vi "IPC-Modbus-Transfer-EncodeResponse-ReadCoils.vi"(11 "Coil Status":bool[](array[boolean])) -> (3 "输出字符串":string)   [LabVIEW 2014]
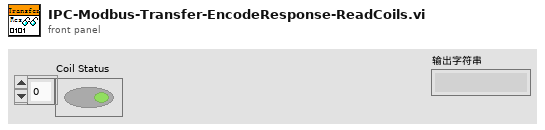
[diagram p1: front panel]
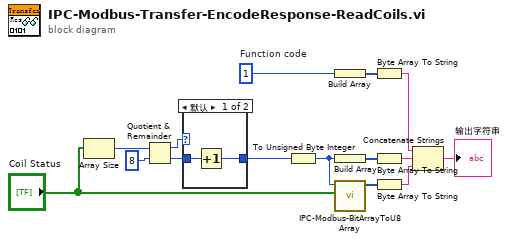
[diagram p0: block diagram]
diagram:
  w10 = u8 1  # Function code
  n1 = Array Size(array="Coil Status") -> (size(s)=w15:i32)
  n2 = Quotient & Remainder(x=w15, y=8) -> (x-y*floor(x/y)=w13:i32, floor(x/y)=w12:i32)
  n3 = case shown="默认" w13 {
    tunnel: w12 -> [w17 w18]
    tunnel: [w16 w18] -> w4
    frame Default {
      n4 = Increment(x=w17) -> (x+1=w16:i32)
    }
    frame 0 {
    }
  }
  n5 = To Unsigned Byte Integer(number=w4) -> (unsigned 8bit integer=w1:u8)
  n6 = Build Array(w10) -> (w11:u8[])
  n7 = Build Array(w1) -> (w9:u8[])
  n8 = call "IPC-Modbus-BitArrayToU8Array.vi"("Bit Array"="Coil Status", "U8 Array size"=w1) -> ("U8 Array"=w2:u8[])  [unwired: 9 in]
  n9 = Byte Array To String(unsigned byte array=w11) -> (string=w8:string)
  n10 = Byte Array To String(unsigned byte array=w9) -> (string=w7:string)
  n11 = Byte Array To String(unsigned byte array=w2) -> (string=w6:string)
  n12 = Concatenate Strings(w8, w7, w6) -> (→"输出字符串":string)
